vi "RetrieveDevicesDB.vi"(8 "error in (no error)":errorcluster, 11 "DatabaseConnectionInfo":T1) -> (0 "error out":errorcluster, 3 "Array":string[][](array[string]))   [LabVIEW 2017]
uses:
  <vilib>/addons/database/Connection.llb/DB Tools Open Connec (Path).vi
  <vilib>/addons/database/_DB Variant To Data/Database Variant To Data.xnode
  <vilib>/addons/database/NI_Database_API.lvlib
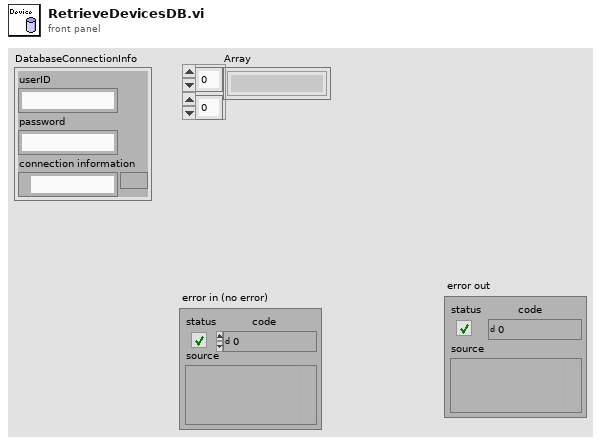
[diagram p1: front panel]
types:
  T1 = cluster{"userID":string, "password":string, "connection information":path}
  T2 = typedef "NI_Database_API.lvlib/Conn ObjectReference.ctl" = refnum<k1>
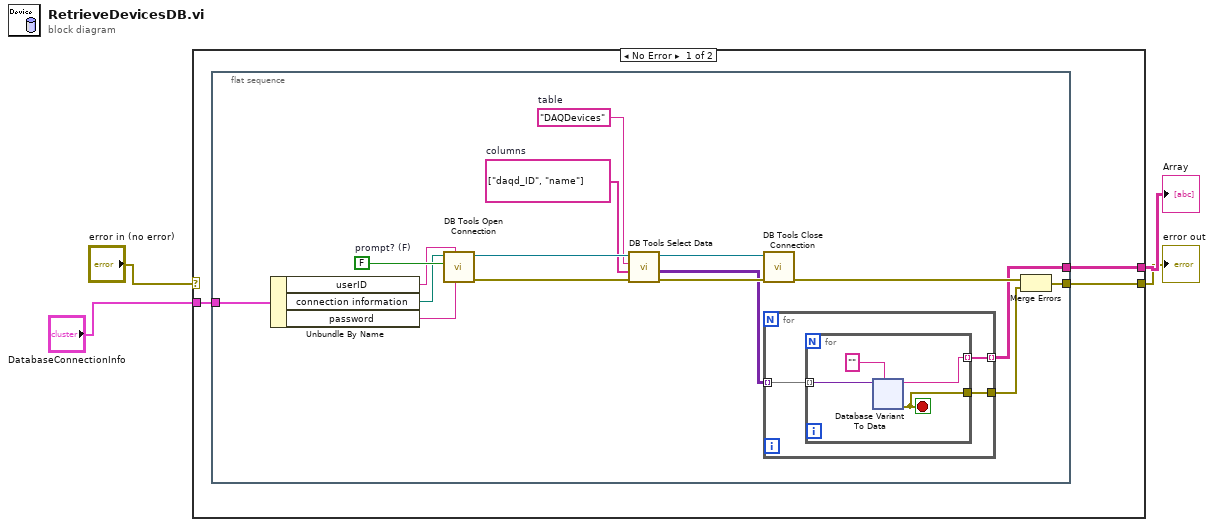
[diagram p0: block diagram]
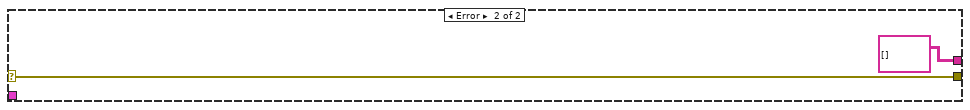
[diagram p2: hidden frame]
diagram:
  n1 = case shown="No Error" "error in (no error)" {
    selector: "error in (no error)" -> [_ w64]
    tunnel: [w7 string[][] []] -> w4
    tunnel: "DatabaseConnectionInfo" -> [w6 _]
    tunnel: [w5 w64] -> w1
    frame No Error {
      n2 = flat-sequence {
        tunnel: [w13] -> w5
        tunnel: [w12] -> w7
        tunnel: w6 -> [w11]
        frame #0 {
          w17 = string[] ["daqd_ID", "name"]  # columns
          w18 = "DAQDevices"  # table
          w23 = FALSE  # prompt? (F)
          n3 = Unbundle By Name(w11) -> ("userID"=w10:string, "connection information"=w8:path, "password"=w9:string)
          n4 = call-poly <vilib>:"DB Tools Open Connection.vi"("password"=w9, "userID"=w10, "prompt? (F)"=w23, "connection information"=w8) -> ("error out"=w21:errorcluster, "connection reference"=w20:T2)  [unwired: 4 in]
          n5 = call <vilib>:"DB Tools Select Data.vi"("error in (no error)"=w21, "columns"=w17, "table"=w18, "connection reference"=w20) -> ("error out"=w19:errorcluster, "data"=w16:variant[][], "connection reference out"=w22:T2)  [unwired: 2 in]
          n6 = call <vilib>:"DB Tools Close Connection.vi"("error in (no error)"=w19, "connection reference"=w22) -> ("error out"=w15:errorcluster)  [unwired: 5 in]
          n7 = for {
            tunnel: w16 -> [w26] mode=indexing
            tunnel: [w25] -> w14
            tunnel: [w24] -> w12 mode=indexing
            n8 = for {
              tunnel: w26 -> [w30] mode=indexing
              tunnel: [w28] -> w25
              tunnel: [w27] -> w24 mode=indexing
              stop <- w28 stop-if-true
              n9 = xnode "Database Variant To Data"("database variant"=w30, "type"="") -> ("data"=w27:string, "error out"=w28:errorcluster)  [unwired: 1 in]
            }
          }
          n10 = Merge Errors(w15, w14) -> (w13:errorcluster)
        }
      }
    }
    frame Error {
    }
  }
  "Array" <- w4
  "error out" <- w1
